vi "Fetch_chirp_waveform_timing.vi"(8 "error in (no error)":errorcluster, 9 "Maximum Time (10000ms)":u32=10000, 10 "Channel (0:Channel1)":u16(ring) items=["Channel1", "Channel2", "Channel3", "Channel4", "Math1", "Math2", "Math3", "Math3", "Reference1", "Reference2", "Reference3", "Reference4"], 11 "VISA resource name":refnum<visa-resource-name>) -> (0 "error out":errorcluster, 1 "meas time":u32, 2 "Waveform Data":waveform(dbl)(graph)={"t0"=timestamp(3.694502999999883e-07 s since 1904-01-01), "dt"=5e-07, "Y"=array[10000 elements]}, 3 "VISA resource name out":refnum<visa-resource-name>, 4 "curve & length command":u32)   [LabVIEW 2011]
doc: "Returns the waveform that an oscilloscope acquires for a channel you specify. An acquisition that you initiate before calling this VI generates the waveform.\n\nYou first enable channels with the Configure Channel VI. Then you use the Initiate VI to start an acquisition on the enabled channels. An oscilloscope concurrently acquires waveforms for these channels. You must call the Fetch Waveform VI separately to obtain waveforms for each enabled channel. However, you also can call the Read Waveform VI instead of using the above low-level VIs.\n\n<B>Note:</B> Use the Fetch Waveform VI only with other low-level VIs, such as the Initiate VI, the Abort VI, and the Fetch Waveform Measurement VI. High-level VIs such as the Read Waveform VI automatically incorporate the functions of the Initiate VI and the Fetch Waveform VI. The Fetch Waveform VI does not check the status of an instrument."
uses:
  <instrlib>/Tektronix 7000 Series/Tektronix 7000 Series.lvlib
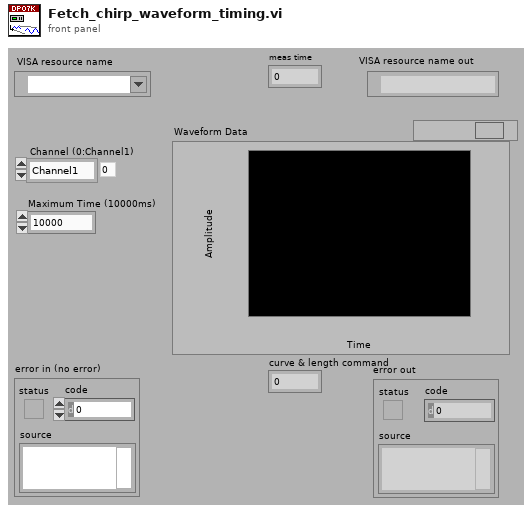
[diagram p1: front panel]
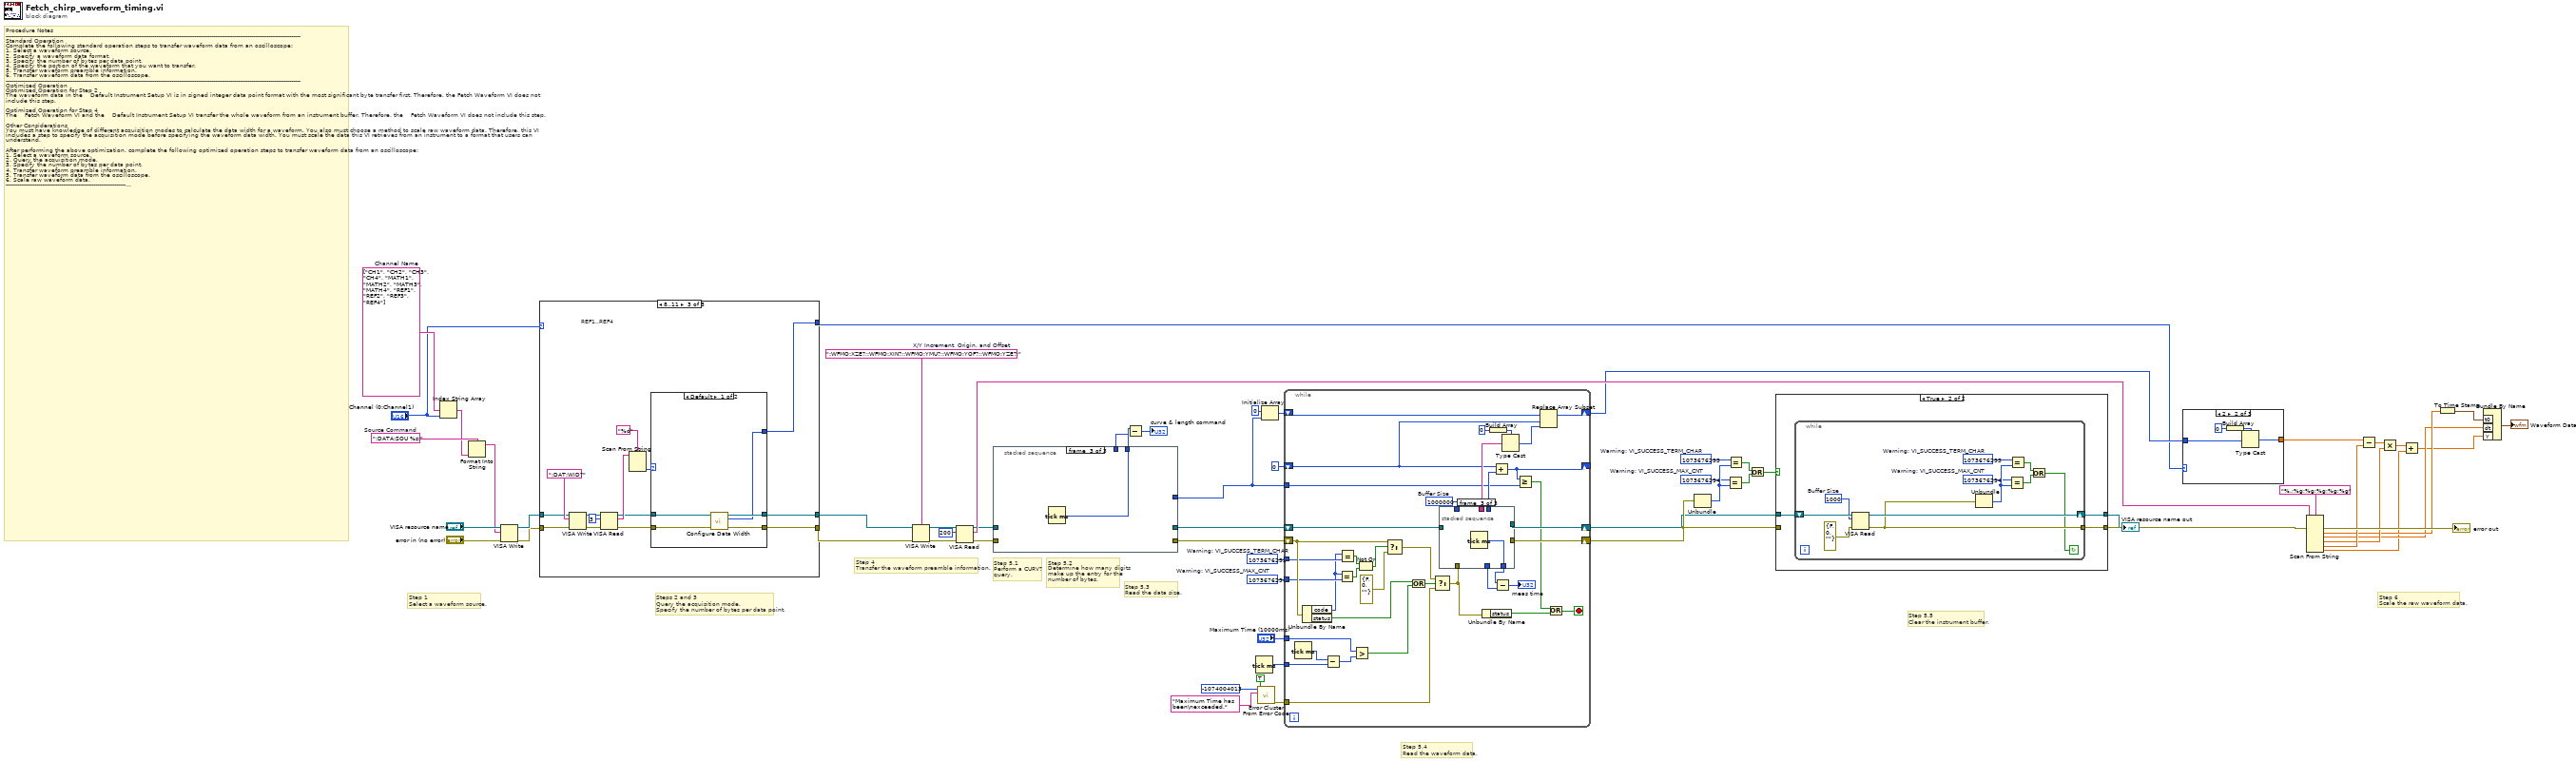
[diagram p0: block diagram]
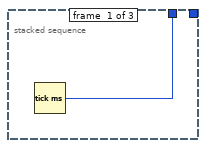
[diagram p2: hidden frame]
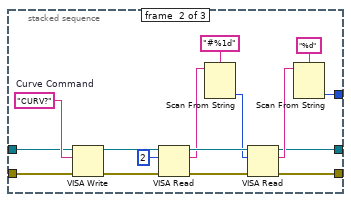
[diagram p3: hidden frame]
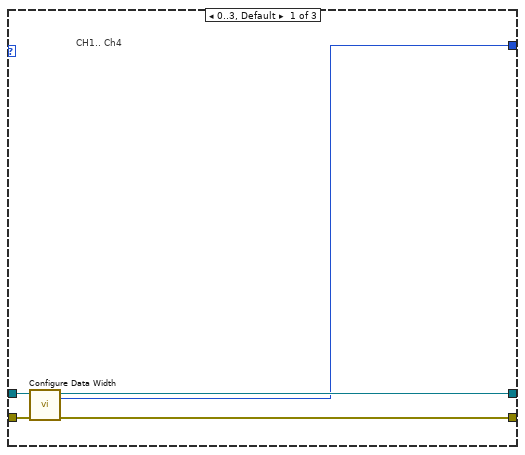
[diagram p4: hidden frame]
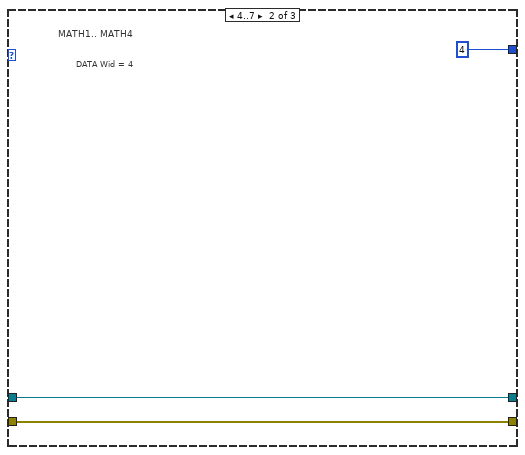
[diagram p5: hidden frame]
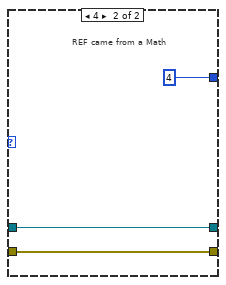
[diagram p6: hidden frame]
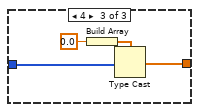
[diagram p8: hidden frame]
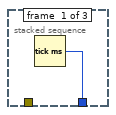
[diagram p10: hidden frame]
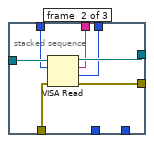
[diagram p11: hidden frame]
diagram:
  w34 = string[] ["CH1", "CH2", "CH3", "CH4", "MATH1", "MATH2", "MATH3", "MATH4", "REF1", "REF2", "REF3", "REF4"]  # Channel Name
  w40 = 1073676294  # Warning: VI_SUCCESS_MAX_CNT
  w41 = 1073676293  # Warning: VI_SUCCESS_TERM_CHAR
  w44 = 1073676294  # Warning: VI_SUCCESS_MAX_CNT
  w43 = 1073676293  # Warning: VI_SUCCESS_TERM_CHAR
  w60 = ":DATA:SOU %s;"  # Source Command
  w29 = ":WFMO:XZE?;:WFMO:XIN?;:WFMO:YMU?;:WFMO:YOF?;:WFMO:YZE?;"  # X/Y Increment, Origin, and Offset
  # "Step 1       \nSelect a waveform source."
  # "Steps 2 and 3\nQuery the acquisition mode. \nSpecify the number of bytes per data point."
  # "Step 6    \nScale the raw waveform data."
  # "Step 5.5    \nClear the instrument buffer."
  # "Step 5.4   \nRead the waveform data."
  # "Step 5.3      \nRead the data size."
  # "Step 5.2      \nDetermine how many digits\nmake up the entry for the \nnumber of bytes."
  # "Step 5.1      \nPerform a CURV?\nquery."
  # "Step 4\nTransfer the waveform preamble information."
  # "Procedure Notes\n-----------------------------------------------------------------------------------------------------------------------------------------------------------\nStandard Operation\nComplete the following standard operation steps to transfer waveform data from an oscilloscope:\n1. Select a waveform source.\n2. Specify a waveform data format.\n3. Specify the number of bytes per data point.\n4. Specify the portion of the waveform that you want to transfer.\n5. Transfer waveform preamble information.\n6. Transfer waveform data from the oscilloscope.\n-----------------------------------------------------------------------------------------------------------------------------------------------------------\nOptimized Operation\nOptimized Operation for Step 2\nThe waveform data in the    Default Instrument Setup VI is in signed integer data point format with the most significant byte transfer first. Therefore, the Fetch Waveform VI does not include this step.\n\nOptimized Operation for Step 4 \nThe    Fetch Waveform VI and the    Default Instrument Setup VI transfer the whole waveform from an instrument buffer. Therefore, the    Fetch Waveform VI does not include this step.\n\nOther Considerations\nYou must have knowledge of different acquisition modes to calculate the data width for a waveform. You also must choose a method to scale raw waveform data. Therefore, this VI includes a step to specify the acquisition mode before specifying the waveform data width. You must scale the data this VI retrieves from an instrument to a format that users can understand.\n\nAfter performing the above optimization, complete the following optimized operation steps to transfer waveform data from an oscilloscope:\n1. Select a waveform source.\n2. Query the acquisition mode.\n3. Specify the number of bytes per data point.\n4. Transfer waveform preamble information.\n5. Transfer waveform data from the oscilloscope.\n6. Scale raw waveform data.\n-----------------------------------------------------------------------------------------------------------------------------------------------------------\nDetailed Steps\nThe following steps detail the behavior of this VI:\n1. Select a waveform source. \n2. Query and determine the acquisition mode. A correct determination is critical to steps 3 and 6.\n    -----------------------------------------------\n    Acquisition Mode |  Data Width   \n    -----------------------------------------------\n    Normal                       |   1                      \n    -----------------------------------------------\n    Peak Detect               |   1                      \n    -----------------------------------------------\n    Hi Res                        |   2                      \n    -----------------------------------------------\n    Envelope                   |   1                      \n    ----------------------------------------------- \n    Average                    |   2                      \n    -----------------------------------------------\n3. Specify the number of bytes per data point. For the Hi Res or Average acquisition modes, set the data width to 2. For all other acquisition modes, set the data width to 1.\n4. Transfer the waveform preamble information. Necessary preamble information includes XZero, XIncrement, YMultiplier, YOffset, and YZero. This VI uses XZero and XIncrement to configure the x-axis of output waveforms and uses YMultiplier, YOffset, and YZero to scale data values. This VI then parses the return string of the preamble query in step 6.\n5. Transfer waveform data from the oscilloscope.\n    5.1 Perform a CURV? query.\n    5.2 Determine how many digits make up the entry for the number of bytes.\n    5.3 Read the data size.\n    5.4 Call the VISA Read VI repeatedly with a buffer size of 10000 until you obtain as much data as the data size specifies. Use      an 8-bit array to store the raw waveform data you obtain. \n    5.5 Continue reading the data remaining in the instrument buffer until the buffer is empty.\n6. Scale the raw waveform data.\n    6.1 Cast the waveform data to a 16-bit array if the data width is 2. Split the waveform data into a minimum and a maximum data array if the acquisition mode is Peak Detect or Envelope. This VI skips this step if the data width is 1.\n    6.2 Parse the preamble information.\n    6.3 Scale the waveform data according to the following formula:\n          Data_Value_in_units = (Raw_Data_Value - YOffset) * YMultiplier + YZero\n          The resulting waveform data has a unit of volts.\n    6.4 Build a waveform graph."
  n1 = Index String Array(1:"Channel (0:Channel1)", 2:w34) -> (0:w59:string)  [unwired: 1 in]
  n2 = Format Into String(format string=w60, w59) -> (resulting string=w31:string)  [unwired: 2 in, 1 out]
  n3 = VISA Write(VISA resource name="VISA resource name", write buffer=w31, error in (no error)="error in (no error)") -> (VISA resource name out=w23:refnum<visa-resource-name>, error out=w22:errorcluster)  [unwired: 1 out]
  n4 = case shown="8..11" "Channel (0:Channel1)" {
    tunnel: w23 -> [w65 w68 w77]
    tunnel: w22 -> [w64 w67 w78]
    tunnel: [w63 w68 w71] -> w5
    tunnel: [w62 w67 w70] -> w4
    tunnel: [w61 u32 4 ("byte count") w69] -> w8
    frame 0..3, Default {
      # "CH1.. Ch4"
      n5 = call <instrlib>:"Configure Data Width.vi"("error in (no error)"=w64, "VISA resource name"=w65) -> ("error out"=w62:errorcluster, "Width"=w61:i32, "VISA resource name out"=w63:refnum<visa-resource-name>)  [unwired: 7 in]
    }
    frame 4..7 {
      # "DATA Wid = 4"
      # "MATH1.. MATH4"
    }
    frame 8..11 {
      # "REF1..REF4"
      n6 = VISA Write(VISA resource name=w77, write buffer=":DAT:WID?", error in (no error)=w78) -> (VISA resource name out=w82:refnum<visa-resource-name>, error out=w81:errorcluster)  [unwired: 1 out]
      n7 = VISA Read(VISA resource name=w82, byte count=u32 3, error in (no error)=w81) -> (VISA resource name out=w73:refnum<visa-resource-name>, read buffer=w76:string, error out=w72:errorcluster)  [unwired: 1 out]
      n8 = Scan From String(format string="%d", input string=w76) -> (output 1=w74:i32)  [unwired: 3 in, 3 out]
      n9 = case shown="Default" w74 {
        tunnel: w73 -> [w87 w90]
        tunnel: w72 -> [w86 w89]
        tunnel: [w85 w90] -> w71
        tunnel: [w84 w89] -> w70
        tunnel: [w83 u32 4 ("byte count")] -> w69
        frame Default {
          n10 = call <instrlib>:"Configure Data Width.vi"("error in (no error)"=w86, "VISA resource name"=w87) -> ("error out"=w84:errorcluster, "Width"=w83:i32, "VISA resource name out"=w85:refnum<visa-resource-name>)  [unwired: 7 in]
        }
        frame 4 {
          # "REF came from a Math"
        }
      }
    }
  }
  n11 = VISA Write(VISA resource name=w5, write buffer=w29, error in (no error)=w4) -> (VISA resource name out=w57:refnum<visa-resource-name>, error out=w56:errorcluster)  [unwired: 1 out]
  n12 = VISA Read(VISA resource name=w57, byte count=u32 200, error in (no error)=w56) -> (VISA resource name out=w21:refnum<visa-resource-name>, read buffer=w55:string, error out=w20:errorcluster)  [unwired: 1 out]
  n13 = stacked-sequence {
    tunnel: [_ w97 _] -> w51
    tunnel: w21 -> [_ w95 _]
    tunnel: w20 -> [_ w94 _]
    tunnel: [_ w93 _] -> w19
    tunnel: [_ w92 _] -> w18
    tunnel: [w91 _ _] -> w2
    tunnel: [_ _ w108] -> w3
    frame #0 {
      n14 = Tick Count (ms)() -> (millisecond timer value=w91:u32)
    }
    frame #1 {
      w107 = "CURV?"  # Curve Command
      n15 = VISA Write(VISA resource name=w95, write buffer=w107, error in (no error)=w94) -> (VISA resource name out=w96:refnum<visa-resource-name>, error out=w106:errorcluster)  [unwired: 1 out]
      n16 = VISA Read(VISA resource name=w96, byte count=u32 2, error in (no error)=w106) -> (VISA resource name out=w103:refnum<visa-resource-name>, read buffer=w101:string, error out=w102:errorcluster)  [unwired: 1 out]
      n17 = Scan From String(format string="#%1d", input string=w101) -> (output 1=w100:i32)  [unwired: 3 in, 3 out]
      n18 = VISA Read(VISA resource name=w103, byte count=w100, error in (no error)=w102) -> (VISA resource name out=w93:refnum<visa-resource-name>, read buffer=w98:string, error out=w92:errorcluster)  [unwired: 1 out]
      n19 = Scan From String(format string="%d", input string=w98) -> (output 1=w97:i32)  [unwired: 3 in, 3 out]
    }
    frame #2 {
      n20 = Tick Count (ms)() -> (millisecond timer value=w108:u32)
    }
  }
  n21 = Subtract(x=w3, y=w2) -> (x-y=→"curve & length command":u32)
  n22 = Tick Count (ms)() -> (millisecond timer value=w11:u32)
  n23 = call <vilib>:"Error Cluster From Error Code.vi"("show call chain? (False)"=TRUE, "error message (\"\")"="Maximum Time has been\nexceeded." ("error message (\"\")"), "error code (0)"=-1074004013) -> ("error out"=w9:errorcluster)  [unwired: 6 in]
  n24 = Initialize Array(i8 0 ("element"), w51) -> (w49:i8[])
  n25 = while {
    shift-right: [w144] -> w6
    shift-left: w19 -> [w146]
    shift-right: [w143] -> w7
    shift-left: w18 -> [w132]
    shift-right: [w139] -> w39
    shift-left: w49 -> [w140]
    tunnel: w51 -> [w136]
    shift-right: [w133] -> _
    shift-left: 0 -> [w134]
    tunnel: w41 -> [w131]
    tunnel: w40 -> [w130]
    tunnel: w11 -> [w124]
    tunnel: "Maximum Time (10000ms)" -> [w123]
    tunnel: w9 -> [w118]
    stop <- w114 stop-if-true
    w145 = 1000000  # Buffer Size
    n26 = Tick Count (ms)() -> (millisecond timer value=w125:u32)
    n27 = Unbundle By Name(w132) -> ("code"=w129:i32, "status"=w117:bool)
    n28 = Subtract(x=w125, y=w124) -> (x-y=w122:u32)
    n29 = Equal?(x=w129, y=w130) -> (x = y?=w127:bool)
    n30 = Equal?(x=w129, y=w131) -> (x = y?=w128:bool)
    n31 = Greater?(x=w123, y=w122) -> (0:w116:bool)
    n32 = Not Or(1:w127, 2:w128) -> (0:w126:bool)
    n33 = Select(t=w132, s=w126, f=errorcluster {"status"=FALSE, "code"=0, "source"=""} ("error in (no error)")) -> (s? t:f=w119:errorcluster)
    n34 = Or(x=w117, y=w116) -> (x .or. y?=w120:bool)
    n35 = Select(t=w119, s=w120, f=w118) -> (s? t:f=w113:errorcluster)
    n36 = stacked-sequence {
      tunnel: w146 -> [_ w154 _]
      tunnel: w145 -> [_ w153 _]
      tunnel: [_ w152 _] -> w144
      tunnel: [_ w151 _] -> w143
      tunnel: [_ w150 _] -> w138
      tunnel: [_ w149 _] -> w137
      tunnel: w113 -> [_ w148 _]
      tunnel: [w147 _ _] -> w110
      tunnel: [_ _ w155] -> w111
      frame #0 {
        n37 = Tick Count (ms)() -> (millisecond timer value=w147:u32)
      }
      frame #1 {
        n38 = VISA Read(VISA resource name=w154, byte count=w153, error in (no error)=w148) -> (VISA resource name out=w152:refnum<visa-resource-name>, read buffer=w150:string, return count=w149:u32, error out=w151:errorcluster)
      }
      frame #2 {
        n39 = Tick Count (ms)() -> (millisecond timer value=w155:u32)
      }
    }
    n40 = Unbundle By Name(w113) -> ("status"=w112:bool)
    n41 = Build Array(i8 0) -> (w142:i8[])
    n42 = Add(x=w134, y=w137) -> (x+y=w133:u32)
    n43 = Subtract(x=w111, y=w110) -> (x-y=→"meas time":u32)
    n44 = Type Cast(type=w142, x=w138) -> (*(type *) &x=w135:i8[])
    n45 = Greater Or Equal?(x=w133, y=w136) -> (x >= y?=w115:bool)
    n46 = Replace Array Subset(array=w140, new element=w135, index=w134) -> (w139:i8[])
    n47 = Or(x=w115, y=w112) -> (x .or. y?=w114:bool)
  }
  n48 = Unbundle(w7) -> ("code"=w45:i32)  [unwired: 2 out]
  n49 = Equal?(x=w44, y=w45) -> (x = y?=w47:bool)
  n50 = Equal?(x=w43, y=w45) -> (x = y?=w48:bool)
  n51 = Or(x=w48, y=w47) -> (x .or. y?=w46:bool)
  n52 = case shown="True" w46 {
    tunnel: w6 -> [w157 w160]
    tunnel: w7 -> [w156 _]
    tunnel: [w157 w159] -> w52
    tunnel: [w156 w158] -> w54
    frame False {
    }
    frame True {
      n53 = while {
        shift-right: [w170] -> w159
        shift-left: w160 -> [w171]
        tunnel: [w163] -> w158
        stop <- w162 continue-if-true
        w165 = 1073676294  # Warning: VI_SUCCESS_MAX_CNT
        w164 = 1073676293  # Warning: VI_SUCCESS_TERM_CHAR
        w169 = u32 1000  # Buffer Size
        n54 = VISA Read(VISA resource name=w171, byte count=w169, error in (no error)=errorcluster {"status"=FALSE, "code"=0, "source"=""}) -> (VISA resource name out=w170:refnum<visa-resource-name>, error out=w163:errorcluster)  [unwired: 2 out]
        n55 = Unbundle(w163) -> ("code"=w166:i32)  [unwired: 2 out]
        n56 = Equal?(x=w165, y=w166) -> (x = y?=w167:bool)
        n57 = Equal?(x=w164, y=w166) -> (x = y?=w168:bool)
        n58 = Or(x=w168, y=w167) -> (x .or. y?=w162:bool)
      }
    }
  }
  "VISA resource name out" <- w52
  n59 = case shown="2" w8 {
    tunnel: w39 -> [w172 w174 w178]
    tunnel: [w172 w173 w177] -> w27
    frame 1, Default {
    }
    frame 2 {
      n60 = Build Array(i16 0 ("element")) -> (w175:i16[])
      n61 = Type Cast(type=w175, x=w174) -> (*(type *) &x=w173:i16[])
    }
    frame 4 {
      n62 = Build Array(sgl 0.0 ("element")) -> (w179:sgl[])
      n63 = Type Cast(type=w179, x=w178) -> (*(type *) &x=w177:sgl[])
    }
  }
  n64 = Scan From String(format string="%.;%g;%g;%g;%g;%g", input string=w55, error in=w54) -> (error out=→"error out":errorcluster, output 1=w26:dbl, output 2=w24:dbl, output 3=w35:dbl, output 4=w36:dbl, output 5=w16:dbl)  [unwired: 6 in, 2 out]
  n65 = Subtract(x=w27, y=w36) -> (x-y=w37:dbl[])
  n66 = Multiply(x=w37, y=w35) -> (x*y=w17:dbl[])
  n67 = Add(x=w17, y=w16) -> (x+y=w15:dbl[])
  n68 = To Time Stamp(1:w26) -> (0:w25:timestamp)
  n69 = Bundle By Name ("Build Waveform")("t0"=w25, "dt"=w24, "Y"=w15) -> (→"Waveform Data":waveform(dbl))  [unwired: 1 in]
